vi "Query Status Register.vi"(8 "error in":errorcluster, 11 "3300 in":refnum<class "3300.lvclass">) -> (0 "error out":errorcluster, 3 "3300 out":refnum<class "3300.lvclass">)   [LabVIEW 2019, in "3300.lvlib" / "3300.lvclass"]
doc: "For the 3300, status register queries are built into the query output routine. \nThis is done because we are sweeping across multiple channels and the 3300 has a 20 ms per command overhead. (meaning if we sweep channels for register, and sweep a second time for measurement we would double the process time for the queries. ie: we do this to speed up the telemetry capabilities of the 3300)"
uses:
  Library/3300.lvclass
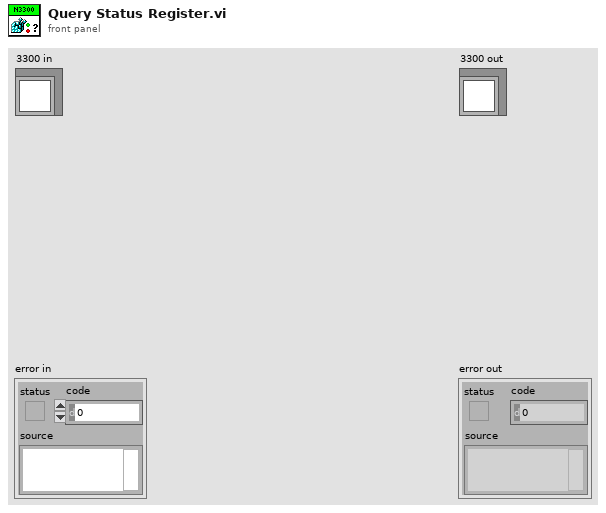
[diagram p1: front panel]
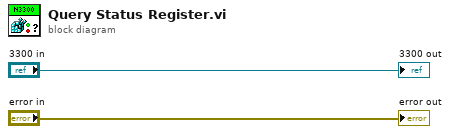
[diagram p0: block diagram]
diagram:
  "error out" <- "error in"
  "3300 out" <- "3300 in"
